vi "Dialog Browse For Folder.vi"(6 "Flags":T1={"return only fs dirs"=FALSE, "don't go below domain"=FALSE, "status text"=FALSE, "return ancestors"=FALSE, "edit box"=TRUE, "validate"=FALSE, "new dialog style"=TRUE, "browse include urls"=FALSE, "browse for computer"=FALSE, "browse for printer"=FALSE, "include files"=FALSE, "sharable"=FALSE, "no new folder button"=FALSE, "no translate targets"=FALSE}, 8 "error in":errorcluster, 10 "Root directory":path, 11 "Title":string) -> (0 "error out":errorcluster, 1 "cancelled":bool, 2 "Selected Path":path)   [LabVIEW 2017, in "OutputToFilePlugins.lvlib" / "OutputToFileBasePlugin.lvclass"]
uses:
  Modules/OutputToFilePlugins/OutputToFileBasePlugin/OutputToFileBasePlugin.lvclass
  shell32.dll
  user32.dll
  kernel32.dll
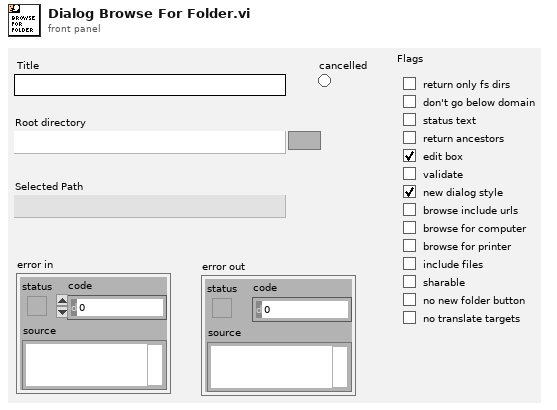
[diagram p1: front panel]
types:
  T1 = cluster{"return only fs dirs":bool, "don't go below domain":bool, "status text":bool, "return ancestors":bool, "edit box":bool, "validate":bool, "new dialog style":bool, "browse include urls":bool, "browse for computer":bool, "browse for printer":bool, "include files":bool, "sharable":bool, "no new folder button":bool, "no translate targets":bool}
  T2 = enum16{"Desktop", "Internet", "Programs", "Control Panel", "Printers", "Personal", "Favorites", "Startup", "Recent", "Sendto", "Bitbucket", "Startmenu", "<undefined 1>", "<undefined 2>", "<undefined 3>", "<undefined 4>", "Desktop Directory", "Drives", "Network", "Nethood", "Fonts", "Templates", "Common Startmenu", "Common Programs", "Common Startup", "Common Desktop Directory", "AppData", "Printhood", "<undefined 5>", "AltStartup", "Common Altstartup", "Common Favorites", "Internet Cache", "Cookies", "History"}
  T3 = cluster{"hWndOwner":u32, "pidlRoot":i32, "pszDisplayName":i32, "lpszTitle":i32, "ulFlags":u32, "lpfn":i32, "lParam":i32, "iImage":i32}
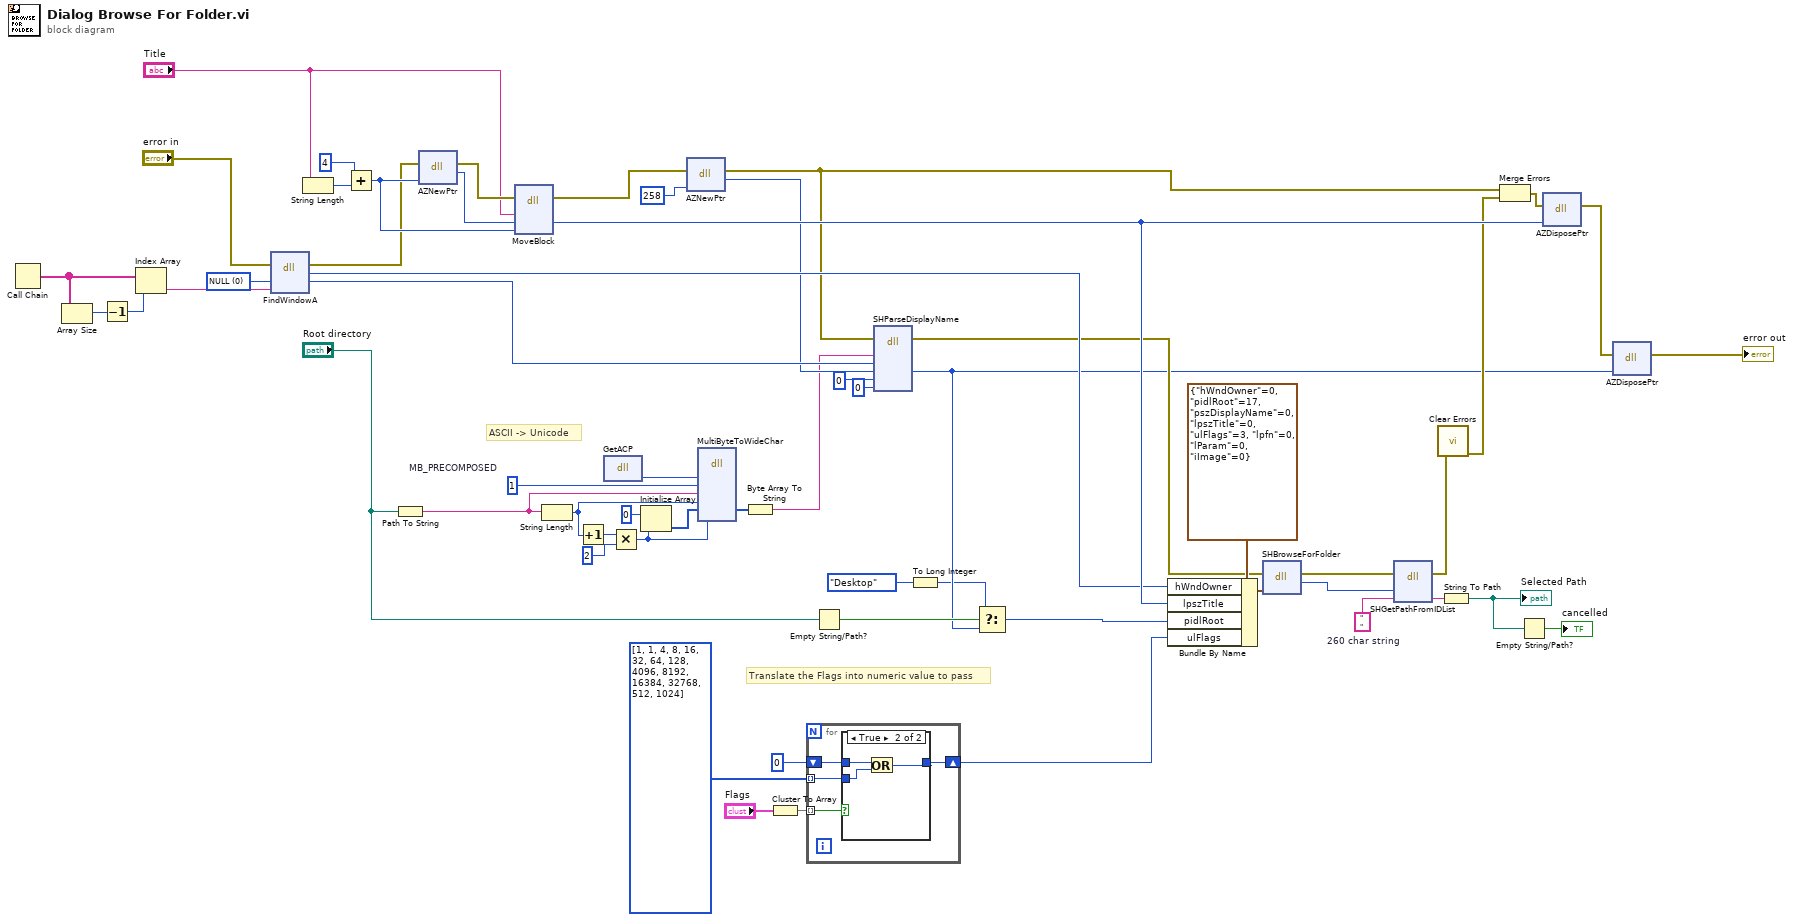
[diagram p0: block diagram]
diagram:
  w9 = u32 1  # MB_PRECOMPOSED
  w39 = 0 items=["NULL"]
  w56 = "                                                                                                                                                                                                                                                                    "  # 260 char string
  # "Translate the Flags into numeric value to pass"
  # "ASCII -> Unicode"
  n1 = Call Chain() -> (call chain=w33:string[])
  n2 = Array Size(array=w33) -> (size(s)=w34:i32)
  n3 = Decrement(x=w34) -> (x-1=w35:i32)
  n4 = Index Array(array=w33, index=w35) -> (element=w32:string)
  n5 = dll-call lib="user32.dll" fn="FindWindowA" label="FindWindow"(error in="error in", "lpszClassName"=w39, "lpszWindowName"=w32) -> (error out=w28:errorcluster, "hWnd"=w44:u32)  [unwired: 4 in, 1 out]
  n6 = String Length(string="Title") -> (length=w50:i32)
  n7 = Add(x=4, y=w50) -> (x+y=w48:i32)
  n8 = Path To String(path="Root directory") -> (string=w7:string)
  n9 = dll-call lib="LabVIEW" fn="AZNewPtr"(error in=w28, "size"=w48) -> (error out=w52:errorcluster, "return type"=w49:i32)  [unwired: 3 in, 1 out]
  n10 = dll-call lib="LabVIEW" fn="MoveBlock"(error in=w52, "src"="Title", "dst"=w49, "size"=w48) -> (error out=w27:errorcluster, "dst"=w46:i32)  [unwired: 4 in, 2 out]
  n11 = String Length(string=w7) -> (length=w14:i32)
  n12 = Increment(x=w14) -> (x+1=w10:i32)
  n13 = dll-call lib="kernel32.dll" fn="GetACP" label="GetACP()"() -> (w16:u32)  [unwired: 3 in, 2 out]
  n14 = Multiply(x=w10, y=2) -> (x*y=w15:i32)
  n15 = Initialize Array(u8 0, w15) -> (w12:u8[])
  n16 = dll-call lib="LabVIEW" fn="AZNewPtr"(error in=w27, "size"=258) -> (error out=w26:errorcluster, "return type"=w36:i32)  [unwired: 3 in, 1 out]
  n17 = dll-call lib="kernel32.dll" fn="MultiByteToWideChar"("codePage"=w16, "dwFlags"=w9, "lpCStr"=w7, "nChars"=w14, "lpWStr"=w12, "nWStr"=w15) -> ("lpWStr"=w13:u8[])  [unwired: 8 in, 3 out]
  n18 = Byte Array To String(unsigned byte array=w13) -> (string=w6:string)
  n19 = Cluster To Array(cluster="Flags") -> (array=w4:bool[])
  n20 = for {
    shift-right: [w59] -> w1
    shift-left: u32 0 ("ulFlags") -> [w60]
    tunnel: w4 -> [w61] mode=indexing
    tunnel: u32[] [1, 1, 4, 8, 16, 32, 64, 128, 4096, 8192, 16384, 32768, 512, 1024] -> [w58] mode=indexing
    n21 = case shown="True" w61 {
      tunnel: w60 -> [w62 w65]
      tunnel: [w62 w64] -> w59
      tunnel: w58 -> [_ w63]
      frame False {
      }
      frame True {
        n22 = Or(x=w65, y=w63) -> (x .or. y?=w64:u32)
      }
    }
  }
  n23 = Empty String/Path?(string/path="Root directory") -> (empty?=w24:bool)
  n24 = dll-call lib="SHELL32.DLL" fn="SHParseDisplayName"(error in=w26, "pszName"=w6, "pbc"=w39, "ppidl"=w36, "sfgaoIn"=u32 0, "psfgaoOut"=u32 0) -> (error out=w25:errorcluster, "ppidl"=w23:i32)  [unwired: 5 in, 3 out]
  n25 = To Long Integer(number=T2."Desktop" ("root")) -> (32bit integer=w20:i32)
  n26 = Select(t=w20, s=w24, f=w23) -> (s? t:f=w22:i32)
  n27 = Bundle By Name(cluster=T3 {"hWndOwner"=0, "pidlRoot"=17, "pszDisplayName"=0, "lpszTitle"=0, "ulFlags"=3, "lpfn"=0, "lParam"=0, "iImage"=0} ("BROWSEINFO"), "hWndOwner"=w44, "lpszTitle"=w46, "pidlRoot"=w22, "ulFlags"=w1) -> (w53:T3)
  n28 = dll-call lib="SHELL32.DLL" fn="SHBrowseForFolder"(error in=w25, "BROWSEINFO"=w53) -> (error out=w45:errorcluster, "PointerToIDList"=w57:i32)  [unwired: 3 in, 1 out]
  n29 = dll-call lib="SHELL32.DLL" fn="SHGetPathFromIDList"(error in=w45, "PointerToIDList"=w57, "PathBuffer"=w56) -> (error out=w41:errorcluster, "PathBuffer"=w55:string)  [unwired: 3 in, 2 out]
  n30 = call <vilib>:"Clear Errors.vi"("error in (no error)"=w41) -> ("error out"=w42:errorcluster)  [unwired: 1 in, 5 out]
  n31 = String To Path(string=w55) -> (path=w18:path)
  "Selected Path" <- w18
  n32 = Merge Errors(w26, w42) -> (w43:errorcluster)
  n33 = Empty String/Path?(string/path=w18) -> (empty?=→"cancelled":bool)
  n34 = dll-call lib="LabVIEW" fn="AZDisposePtr"(error in=w43, "pointer"=w46) -> (error out=w30:errorcluster)  [unwired: 3 in, 2 out]
  n35 = dll-call lib="LabVIEW" fn="AZDisposePtr"(error in=w30, "pointer"=w23) -> (error out=→"error out":errorcluster)  [unwired: 3 in, 2 out]
